vi "rsscope_core_global.vi"() -> ()   [LabVIEW 2018] (continued)
 Models"="", "Instrument Options"="K3", "Flags"=0, "Help"="Sets the LIN standard to search for CRC errors.\n\nAvailable Repeated Capabilities:\nNone\n\nRemote-control command(s):\nSEARch:TRIGger:LIN:STANdard"}, {"Level"=5, "Class Only"=FALSE, "Identifier"="RSSCOPE_ATTR_SEARCH_LIN_IDENTIFIER_PARITY_ERROR", "Descriptive Name"="Search LIN Identifier Parity Error", "Data Type"=3, "Command"="SEAR:TRIG:LIN:IPER", "Access"=2, "Range Table"="", "Read Callback"="rsscope_FormatSearchNameBoolean_ReadCallback.vi", "Write Callback"="rsscope_FormatSearchNameBoolean_WriteCallback.vi", "Supported Models"="", "Instrument Options"="K3", "Flags"=0, "Help"="Searches for errors in the identifier parity bits. These are the bits 6 and 7 of the identifier.\n\nAvailable Repeated Capabilities:\nNone\n\nRemote-control command(s):\nSEARch:TRIGger:LIN:IPERror"}, {"Level"=5, "Class Only"=FALSE, "Identifier"="RSSCOPE_ATTR_SEARCH_LIN_SYNC_ERROR", "Descriptive Name"="Search LIN Sync Error", "Data Type"=3, "Command"="SEAR:TRIG:LIN:SYER", "Access"=2, "Range Table"="", "Read Callback"="rsscope_FormatSearchNameBoolean_ReadCallback.vi", "Write Callback"="rsscope_FormatSearchNameBoolean_WriteCallback.vi", "Supported Models"="", "Instrument Options"="K3", "Flags"=0, "Help"="Searches for synchronization errors.\n\nAvailable Repeated Capabilities:\nNone\n\nRemote-control command(s):\nSEARch:TRIGger:LIN:SYERror"}, {"Level"=4, "Class Only"=TRUE, "Identifier"="", "Descriptive Name"="Results", "Data Type"=0, "Command"="", "Access"=0, "Range Table"="", "Read Callback"="", "Write Callback"="", "Supported Models"="", "Instrument Options"="", "Flags"=0, "Help"="Returns the search result of the specified frame."}, {"Level"=5, "Class Only"=FALSE, "Identifier"="RSSCOPE_ATTR_SEARCH_LIN_SELECTED_FRAME", "Descriptive Name"="Search LIN Selected Frame", "Data Type"=0, "Command"="", "Access"=2, "Range Table"="", "Read Callback"="", "Write Callback"="", "Supported Models"="", "Instrument Options"="", "Flags"=0, "Help"="Sets the selector for the Frame repeated capability.\n\nAvailable Repeated Capabilities:\nNone\n\nRemote-control command(s):\n"}, {"Level"=5, "Class Only"=FALSE, "Identifier"="RSSCOPE_ATTR_SEARCH_LIN_FRAME_COUNT", "Descriptive Name"="Search LIN Frame Count", "Data Type"=0, "Command"="SEAR:RES:LIN:FCO?", "Access"=0, "Range Table"="", "Read Callback"="rsscope_FormatSearchNameInt32_ReadCallback.vi", "Write Callback"="", "Supported Models"="", "Instrument Options"="K3", "Flags"=0, "Help"="Returns the frame count for the selected serial bus.\n\nAvailable Repeated Capabilities:\nNone\n\nRemote-control command(s):\nSEARch:RESult:LIN:FCOunt?"}, {"Level"=5, "Class Only"=FALSE, "Identifier"="RSSCOPE_ATTR_SEARCH_LIN_FRAME_SYMBOLIC_DATA", "Descriptive Name"="Search LIN Frame Symbolic Data", "Data Type"=2, "Command"="SEAR:RES:LIN:FRAM<Frame>:SDAT?", "Access"=0, "Range Table"="", "Read Callback"="rsscope_FormatLINSearchNameFrameRepCapString_ReadCallback.vi", "Write Callback"="rsscope_FormatLINSearchNameFrameRepCapString_WriteCallback.vi", "Supported Models"="", "Instrument Options"="", "Flags"=0, "Help"="Returns the symbolic data of the frame.\n\nAvailable Repeated Capabilities:\nNone\n\nRemote-control command(s):\nSEARch:RESult:LIN:FRAMe<m>:SDATa?"}, {"Level"=5, "Class Only"=FALSE, "Identifier"="RSSCOPE_ATTR_SEARCH_LIN_FRAME_SYMBOLIC_DATA_EXPORT", "Descriptive Name"="Search LIN Frame Symbolic Data Export", "Data Type"=2, "Command"="SEAR:RES:LIN:FRAM<Frame>:SDEX?", "Access"=0, "Range Table"="", "Read Callback"="rsscope_FormatLINSearchNameFrameRepCapString_ReadCallback.vi", "Write Callback"="rsscope_FormatLINSearchNameFrameRepCapString_WriteCallback.vi", "Supported Models"="", "Instrument Options"="", "Flags"=0, "Help"="Returns the symbolic data of the frame for the export format.\n\nAvailable Repeated Capabilities:\nNone\n\nRemote-control command(s):\nSEARch:RESult:LIN:FRAMe<m>:SDEXport?"}, {"Level"=3, "Class Only"=TRUE, "Identifier"="", "Descriptive Name"="CAN", "Data Type"=0, "Command"="", "Access"=0, "Range Table"="", "Read Callback"="", "Write Callback"="", "Supported Models"="", "Instrument Options"="", "Flags"=0, "Help"="Search decoded data in CAN protocol."}, {"Level"=4, "Class Only"=FALSE, "Identifier"="RSSCOPE_ATTR_SEARCH_CAN_ENABLED", "Descriptive Name"="Search CAN Enabled", "Data Type"=3, "Command"="SEAR:TRIG:CAN", "Access"=2, "Range Table"="", "Read Callback"="rsscope_FormatSearchNameBoolean_ReadCallback.vi", "Write Callback"="rsscope_FormatSearchNameBoolean_WriteCallback.vi", "Supported Models"="", "Instrument Options"="", "Flags"=0, "Help"="Includes the search conditions for the CAN trigger event type in the next search.\n\nAvailable Repeated Capabilities:\nNone\n\nRemote-control command(s):\nSEARch:TRIGger:CAN[:STATe]"}, {"Level"=4, "Class Only"=FALSE, "Identifier"="RSSCOPE_ATTR_SEARCH_CAN_COPY_FROM_A", "Descriptive Name"="Search CAN Copy From A", "Data Type"=2, "Command"="SEAR:TRIG:CAN:ACOP", "Access"=1, "Range Table"="", "Read Callback"="", "Write Callback"="", "Supported Models"="", "Instrument Options"="", "Flags"=0, "Help"="Copies the trigger event configuration from Trigger A for the selcted CAN bus to the search condition settings.\n\nAvailable Repeated Capabilities:\nNone\n\nRemote-control command(s):\nSEARch:TRIGger:CAN:ACOPy"}, {"Level"=4, "Class Only"=FALSE, "Identifier"="RSSCOPE_ATTR_SEARCH_CAN_START_OF_FRAME_ENABLED", "Descriptive Name"="Search CAN Start Of Frame Enabled", "Data Type"=3, "Command"="SEAR:TRIG:CAN:SSOF", "Access"=2, "Range Table"="", "Read Callback"="rsscope_FormatSearchNameBoolean_ReadCallback.vi", "Write Callback"="rsscope_FormatSearchNameBoolean_WriteCallback.vi", "Supported Models"="", "Instrument Options"="", "Flags"=0, "Help"="Enables the search for a start of frame.\n\nAvailable Repeated Capabilities:\nNone\n\nRemote-control command(s):\nSEARch:TRIGger:CAN[:SSOFrame]"}, {"Level"=4, "Class Only"=FALSE, "Identifier"="RSSCOPE_ATTR_SEARCH_CAN_FRAME_TYPE_ENABLED", "Descriptive Name"="Search CAN Frame Type Enabled", "Data Type"=3, "Command"="SEAR:TRIG:CAN:SFTY", "Access"=2, "Range Table"="", "Read Callback"="rsscope_FormatSearchNameBoolean_ReadCallback.vi", "Write Callback"="rsscope_FormatSearchNameBoolean_WriteCallback.vi", "Supported Models"="", "Instrument Options"="", "Flags"=0, "Help"="Enables the search for a specified frame type.\n\nAvailable Repeated Capabilities:\nNone\n\nRemote-control command(s):\nSEARch:TRIGger:CAN:SFTYpe"}, {"Level"=4, "Class Only"=FALSE, "Identifier"="RSSCOPE_ATTR_SEARCH_CAN_FRAME_IDENTIFIER_ENABLED", "Descriptive Name"="Search CAN Frame Identifier Enabled", "Data Type"=3, "Command"="SEAR:TRIG:CAN:SFID", "Access"=2, "Range Table"="", "Read Callback"="rsscope_FormatSearchNameBoolean_ReadCallback.vi", "Write Callback"="rsscope_FormatSearchNameBoolean_WriteCallback.vi", "Supported Models"="", "Instrument Options"="", "Flags"=0, "Help"="Enables the search for frame indentifier.\n\nAvailable Repeated Capabilities:\nNone\n\nRemote-control command(s):\nSEARch:TRIGger:CAN:SFIDentifier"}, {"Level"=4, "Class Only"=FALSE, "Identifier"="RSSCOPE_ATTR_SEARCH_CAN_IDENTIFIER_DATA_ENABLED", "Descriptive Name"="Search CAN Identifier Data Enabled", "Data Type"=3, "Command"="SEAR:TRIG:CAN:SIDD", "Access"=2, "Range Table"="", "Read Callback"="rsscope_FormatSearchNameBoolean_ReadCallback.vi", "Write Callback"="rsscope_FormatSearchNameBoolean_WriteCallback.vi", "Supported Models"="", "Instrument Options"="", "Flags"=0, "Help"="Enables the search for identifier and data.\n\nAvailable Repeated Capabilities:\nNone\n\nRemote-control command(s):\nSEARch:TRIGger:CAN:SIDData"}, {"Level"=4, "Class Only"=FALSE, "Identifier"="RSSCOPE_ATTR_SEARCH_CAN_SYMBOLIC_ENABLED", "Descriptive Name"="Search CAN Symbolic Enabled", "Data Type"=3, "Command"="SEAR:TRIG:CAN:SSYM", "Access"=2, "Range Table"="", "Read Callback"="rsscope_FormatSearchNameBoolean_ReadCallback.vi", "Write Callback"="rsscope_FormatSearchNameBoolean_WriteCallback.vi", "Supported Models"="", "Instrument Options"="", "Flags"=0, "Help"="Enables the symbolic search and disables all other search criteria.\n\nAvailable Repeated Capabilities:\nNone\n\nRemote-control command(s):\nSEARch:TRIGger:CAN:SSYMbolic"}, {"Level"=4, "Class Only"=FALSE, "Identifier"="RSSCOPE_ATTR_SEARCH_CAN_FRAME_TYPE", "Descriptive Name"="Search CAN Frame Type", "Data Type"=0, "Command"="SEAR:TRIG:CAN:FTYP", "Access"=2, "Range Table"="rsscope_rngProtocolCANTriggFrameType", "Read Callback"="rsscope_FormatSearchNameInt32_ReadCallback.vi", "Write Callback"="rsscope_FormatSearchNameInt32_WriteCallback.vi", "Supported Models"="", "Instrument Options"="", "Flags"=0, "Help"="Selects the CAN frame type to be searched for.\n\nAvailable Repeated Capabilities:\nNone\n\nRemote-control command(s):\nSEARch:TRIGger:CAN:FTYPe"}, {"Level"=4, "Class Only"=FALSE, "Identifier"="RSSCOPE_ATTR_SEARCH_CAN_STANDARD", "Descriptive Name"="Search CAN Standard", "Data Type"=0, "Command"="SEAR:TRIG:CAN:FDAT:STAN", "Access"=2, "Range Table"="rsscope_rngCANStandard", "Read Callback"="rsscope_FormatSearchNameInt32_ReadCallback.vi", "Write Callback"="rsscope_FormatSearchNameInt32_WriteCallback.vi", "Supported Models"="", "Instrument Options"="K9", "Flags"=0, "Help"="Selects the CAN standard: CAN, CAN FD, or Any.\n\nAvailable Repeated Capabilities:\nNone\n\nRemote-control command(s):\nSEARch:TRIGger:CAN:FDATa:STANdard"}, {"Level"=4, "Class Only"=FALSE, "Identifier"="RSSCOPE_ATTR_SEARCH_CAN_ID_TYPE", "Descriptive Name"="Search CAN ID Type", "Data Type"=0, "Command"="SEAR:TRIG:CAN:ITYP", "Access"=2, "Range Table"="rsscope_rngProtocolCANIDType", "Read Callback"="rsscope_FormatSearchNameInt32_ReadCallback.vi", "Write Callback"="rsscope_FormatSearchNameInt32_WriteCallback.vi", "Supported Models"="", "Instrument Options"="", "Flags"=0, "Help"="Selects the format of data and remote frames: 11 bit for CAN base frames, or 29 bits for CAN extended frames.\n\nAvailable Repeated Capabilities:\nNone\n\nRemote-control command(s):\nSEARch:TRIGger:CAN:ITYPe"}, {"Level"=4, "Class Only"=FALSE, "Identifier"="RSSCOPE_ATTR_SEARCH_CAN_IDENTIFIER_CONDITION", "Descriptive Name"="Search CAN Identifier Condition", "Data Type"=0, "Command"="SEAR:TRIG:CAN:ICON", "Access"=2, "Range Table"="rsscope_rngProtocolTriggerCondition", "Read Callback"="rsscope_FormatSearchNameInt32_ReadCallback.vi", "Write Callback"="rsscope_FormatSearchNameInt32_WriteCallback.vi", "Supported Models"="", "Instrument Options"="", "Flags"=0, "Help"="Sets the operator to set a specific identifier or an identifier range.\n\nAvailable Repeated Capabilities:\nNone\n\nRemote-control command(s):\nSEARch:TRIGger:CAN:ICONdition"}, {"Level"=4, "Class Only"=FALSE, "Identifier"="RSSCOPE_ATTR_SEARCH_CAN_IDENTIFIER_MIN", "Descriptive Name"="Search CAN Identifier Min", "Data Type"=2, "Command"="SEAR:TRIG:CAN:IMIN", "Access"=1, "Range Table"="", "Read Callback"="", "Write Callback"="rsscope_FormatSearchNameString_WriteCallback.vi", "Supported Models"="", "Instrument Options"="", "Flags"=0, "Help"="Specifies a message identifier pattern, or sets the start value of an identifier range.\n\nAvailable Repeated Capabilities:\nNone\n\nRemote-control command(s):\nSEARch:TRIGger:CAN:IMIN"}, {"Level"=4, "Class Only"=FALSE, "Identifier"="RSSCOPE_ATTR_SEARCH_CAN_IDENTIFIER_MAX", "Descriptive Name"="Search CAN Identifier Max", "Data Type"=2, "Command"="SEAR:TRIG:CAN:IMAX", "Access"=1, "Range Table"="", "Read Callback"="", "Write Callback"="rsscope_FormatSearchNameString_WriteCallback.vi", "Supported Models"="", "Instrument Options"="", "Flags"=0, "Help"="Sets the end value of an identifier range if RSSCOPE_ATTR_SEARCH_CAN_IDENTIFIER_CONDITION is set to In range or Out of range.\n\nAvailable Repeated Capabilities:\nNone\n\nRemote-control command(s):\nSEARch:TRIGger:CAN:IMAX"}, {"Level"=4, "Class Only"=FALSE, "Identifier"="RSSCOPE_ATTR_SEARCH_CAN_FD_BITS_FDF", "Descriptive Name"="Search CAN FD Bits FDF", "Data Type"=0, "Command"="SEAR:TRIG:CAN:FDAT", "Access"=2, "Range Table"="rsscope_rngCANFDBits", "Read Callback"="rsscope_FormatSearchNameInt32_ReadCallback.vi", "Write Callback"="rsscope_FormatSearchNameInt32_WriteCallback.vi", "Supported Models"="", "Instrument Options"="K9", "Flags"=0, "Help"="Specifies the CAN FD frame format. It corresponds to the EDL bit (extended data length), which only exists in CAN FD format.\n\nAvailable Repeated Capabilities:\nNone\n\nRemote-control command(s):\nSEARch:TRIGger:CAN:FDATa[:FDF]"}, {"Level"=4, "Class Only"=FALSE, "Identifier"="RSSCOPE_ATTR_SEARCH_CAN_FD_BITS_BRS", "Descriptive Name"="Search CAN FD Bits BRS", "Data Type"=0, "Command"="SEAR:TRIG:CAN:FDAT:BRS", "Access"=2, "Range Table"="rsscope_rngCANFDBits", "Read Callback"="rsscope_FormatSearchNameInt32_ReadCallback.vi", "Write Callback"="rsscope_FormatSearchNameInt32_WriteCallback.vi", "Supported Models"="", "Instrument Options"="K9", "Flags"=0, "Help"="Sets the bit rate switch bit.\n\nAvailable Repeated Capabilities:\nNone\n\nRemote-control command(s):\nSEARch:TRIGger:CAN:FDATa:BRS"}, {"Level"=4, "Class Only"=FALSE, "Identifier"="RSSCOPE_ATTR_SEARCH_CAN_FD_BITS_ESI", "Descriptive Name"="Search CAN FD Bits ESI", "Data Type"=0, "Command"="SEAR:TRIG:CAN:FDAT:ESI", "Access"=2, "Range Table"="rsscope_rngCANFDBits", "Read Callback"="rsscope_FormatSearchNameInt32_ReadCallback.vi", "Write Callback"="rsscope_FormatSearchNameInt32_WriteCallback.vi", "Supported Models"="", "Instrument Options"="K9", "Flags"=0, "Help"="Sets the error state indicator bit.\n\nAvailable Repeated Capabilities:\nNone\n\nRemote-control command(s):\nSEARch:TRIGger:CAN:FDATa:ESI"}, {"Level"=4, "Class Only"=FALSE, "Identifier"="RSSCOPE_ATTR_SEARCH_CAN_DLC_CONDITION", "Descriptive Name"="Search CAN DLC Condition", "Data Type"=0, "Command"="SEAR:TRIG:CAN:DLCC", "Access"=2, "Range Table"="rsscope_rngProtocolTriggerCondition", "Read Callback"="rsscope_FormatSearchNameInt32_ReadCallback.vi", "Write Callback"="rsscope_FormatSearchNameInt32_WriteCallback.vi", "Supported Models"="", "Instrument Options"="", "Flags"=0, "Help"="Operator to set the data length code for searching on CAN data. For big endian transfer direction, you can search for a number of bytes less than the DLC of the frame, that means, on the beginning of the data pattern. For little endian transfer direction, the exact number of data bytes in the frame must be set. The number of data bytes to be found is set with RSSCOPE_ATTR_SEARCH_CAN_DLC\n\nAvailable Repeated Capabilities:\nNone\n\nRemote-control command(s):\nSEARch:TRIGger:CAN:DLCCondition"}, {"Level"=4, "Class Only"=FALSE, "Identifier"="RSSCOPE_ATTR_SEARCH_CAN_DLC", "Descriptive Name"="Search CAN DLC", "Data Type"=0, "Command"="SEAR:TRIG:CAN:DLC", "Access"=2, "Range Table"="RsScope_rngSearchCANDLC", "Read Callback"="rsscope_FormatSearchNameInt32_ReadCallback.vi", "Write Callback"="rsscope_FormatSearchNameInt32_WriteCallback.vi", "Supported Models"="", "Instrument Options"="", "Flags"=0, "Help"="Sets the Data Length Code, the number of data bytes to be found. For complete definition, set also the operator with RSSCOPE_ATTR_SEARCH_CAN_DLC_CONDITION.\n\nAvailable Repeated Capabilities:\nNone\n\nRemote-control command(s):\nSEARch:TRIGger:CAN:DLC"}, {"Level"=4, "Class Only"=FALSE, "Identifier"="RSSCOPE_ATTR_SEARCH_CAN_POSITION_CONDITION", "Descriptive Name"="Search CAN Position Condition", "Data Type"=0, "Command"="SEAR:TRIG:CAN:FDAT:DPOP", "Access"=2, "Range Table"="rsscope_rngProtocolCANPositionCondition", "Read Callback"="rsscope_FormatSearchNameInt32_ReadCallback.vi", "Write Callback"="rsscope_FormatSearchNameInt32_WriteCallback.vi", "Supported Models"="", "Instrument Options"="K9", "Flags"=0, "Help"="Sets the operator to define an exact position or a data range where the instrument looks for the specified data pattern.\n\nAvailable Repeated Capabilities:\nNone\n\nRemote-control command(s):\nSEARch:TRIGger:CAN:FDATa:DPOPerator"}, {"Level"=4, "Class Only"=FALSE, "Identifier"="RSSCOPE_ATTR_SEARCH_CAN_POSITION_MIN", "Descriptive Name"="Search CAN Position Min", "Data Type"=0, "Command"="SEAR:TRIG:CAN:FDAT:DPOS", "Access"=2, "Range Table"="rsscope_rngCANPositionMin", "Read Callback"="rsscope_FormatSearchNameInt32_ReadCallback.vi", "Write Callback"="rsscope_FormatSearchNameInt32_WriteCallback.vi", "Supported Models"="", "Instrument Options"="K9", "Flags"=0, "Help"="Defines the first possible start position of the data pattern.\n\nAvailable Repeated Capabilities:\nNone\n\nRemote-control command(s):\nSEARch:TRIGger:CAN:FDATa:DPOSition"}, {"Level"=4, "Class Only"=FALSE, "Identifier"="RSSCOPE_ATTR_SEARCH_CAN_POSITION_MAX", "Descriptive Name"="Search CAN Position Max", "Data Type"=0, "Command"="SEAR:TRIG:CAN:FDAT:DPTO", "Access"=2, "Range Table"="rsscope_rngCANPositionMax", "Read Callback"="rsscope_FormatSearchNameInt32_ReadCallback.vi", "Write Callback"="rsscope_FormatSearchNameInt32_WriteCallback.vi", "Supported Models"="", "Instrument Options"="K9", "Flags"=0, "Help"="Defines the last possible start position of the data pattern if &apos;Condition&apos; is &apos;In range&apos; and &apos;Out of range&apos;.\n\nAvailable Repeated Capabilities:\nNone\n\nRemote-control command(s):\nSEARch:TRIGger:CAN:FDATa:DPTO"}, {"Level"=4, "Class Only"=FALSE, "Identifier"="RSSCOPE_ATTR_SEARCH_CAN_DATA_CONDITION", "Descriptive Name"="Search CAN Data Condition", "Data Type"=0, "Command"="SEAR:TRIG:CAN:DCON", "Access"=2, "Range Table"="rsscope_rngProtocolTriggerCondition", "Read Callback"="rsscope_FormatSearchNameInt32_ReadCallback.vi", "Write Callback"="rsscope_FormatSearchNameInt32_WriteCallback.vi", "Supported Models"="", "Instrument Options"="", "Flags"=0, "Help"="Sets the operator to set a specific data pattern or a data pattern range.\n\nAvailable Repeated Capabilities:\nNone\n\nRemote-control command(s):\nSEARch:TRIGger:CAN:DCONdition"}, {"Level"=4, "Class Only"=FALSE, "Identifier"="RSSCOPE_ATTR_SEARCH_CAN_DATA_MIN", "Descriptive Name"="Search CAN Data Min", "Data Type"=2, "Command"="SEAR:TRIG:CAN:DMIN", "Access"=1, "Range Table"="", "Read Callback"="", "Write Callback"="rsscope_FormatSearchNameString_WriteCallback.vi", "Supported Models"="", "Instrument Options"="", "Flags"=0, "Help"="Specifies a data pattern, or sets the start value of a data pattern range.\n\nAvailable Repeated Capabilities:\nNone\n\nRemote-control command(s):\nSEARch:TRIGger:CAN:DMIN"}, {"Level"=4, "Class Only"=FALSE, "Identifier"="RSSCOPE_ATTR_SEARCH_CAN_DATA_MAX", "Descriptive Name"="Search CAN Data Max", "Data Type"=2, "Command"="SEAR:TRIG:CAN:DMAX", "Access"=1, "Range Table"="", "Read Callback"="", "Write Callback"="rsscope_FormatSearchNameString_WriteCallback.vi", "Supported Models"="", "Instrument Options"="", "Flags"=0, "Help"="Sets the end value of an data range if RSSCOPE_ATTR_SEARCH_CAN_DATA_CONDITION is set to In range or Out of range.\n\nAvailable Repeated Capabilities:\nNone\n\nRemote-control command(s):\nSEARch:TRIGger:CAN:DMAX"}, {"Level"=4, "Class Only"=FALSE, "Identifier"="RSSCOPE_ATTR_SEARCH_CAN_CRC_ERROR", "Descriptive Name"="Search CAN CRC Error", "Data Type"=3, "Command"="SEAR:TRIG:CAN:CRC", "Access"=2, "Range Table"="", "Read Callback"="rsscope_FormatSearchNameBoolean_ReadCallback.vi", "Write Callback"="rsscope_FormatSearchNameBoolean_WriteCallback.vi", "Supported Models"="", "Instrument Options"="", "Flags"=0, "Help"="Searches for errors in the Cyclic Redundancy Check.\n\nAvailable Repeated Capabilities:\nNone\n\nRemote-control command(s):\nSEARch:TRIGger:CAN:CRCerror"}, {"Level"=4, "Class Only"=FALSE, "Identifier"="RSSCOPE_ATTR_SEARCH_CAN_BIT_STUFFING_ERROR", "Descriptive Name"="Search CAN Bit Stuffing Error", "Data Type"=3, "Command"="SEAR:TRIG:CAN:BITS", "Access"=2, "Range Table"="", "Read Callback"="rsscope_FormatSearchNameBoolean_ReadCallback.vi", "Write Callback"="rsscope_FormatSearchNameBoolean_WriteCallback.vi", "Supported Models"="", "Instrument Options"="", "Flags"=0, "Help"="Searches for bit stuffing errors.\n\nAvailable Repeated Capabilities:\nNone\n\nRemote-control command(s):\nSEARch:TRIGger:CAN:BITSterror"}, {"Level"=4, "Class Only"=FALSE, "Identifier"="RSSCOPE_ATTR_SEARCH_CAN_ACK_ERROR", "Descriptive Name"="Search CAN Ack Error", "Data Type"=3, "Command"="SEAR:TRIG:CAN:ACK", "Access"=2, "Range Table"="", "Read Callback"="rsscope_FormatSearchNameBoolean_ReadCallback.vi", "Write Callback"="rsscope_FormatSearchNameBoolean_WriteCallback.vi", "Supported Models"="", "Instrument Options"="", "Flags"=0, "Help"="Searches for acknowledgement errors. An acknowledgement error occurs when the transmitter does not receive an acknowledgment - a dominant bit during the Ack Slot.\n\nAvailable Repeated Capabilities:\nNone\n\nRemote-control command(s):\nSEARch:TRIGger:CAN:ACKerror"}, {"Level"=4, "Class Only"=FALSE, "Identifier"="RSSCOPE_ATTR_SEARCH_CAN_STUFF_COUNT_ERROR", "Descriptive Name"="Search CAN Stuff Count Error", "Data Type"=3, "Command"="SEAR:TRIG:CAN:FDAT:SCER", "Access"=2, "Range Table"="", "Read Callback"="rsscope_FormatSearchNameBoolean_ReadCallback.vi", "Write Callback"="rsscope_FormatSearchNameBoolean_WriteCallback.vi", "Supported Models"="", "Instrument Options"="K3", "Flags"=0, "Help"="Triggers on stuff count errors. A stuff count error occurs if th received stuff count value does not match the value calculated from the own stuff bit count.\n\nAvailable Repeated Capabilities:\nNone\n\nRemote-control command(s):\nSEARch:TRIGger:CAN:FDATa:SCERror"}, {"Level"=4, "Class Only"=TRUE, "Identifier"="", "Descriptive Name"="Symbolic", "Data Type"=0, "Command"="", "Access"=0, "Range Table"="", "Read Callback"="", "Write Callback"="", "Supported Models"="", "Instrument Options"="", "Flags"=0, "Help"="This class configures symbolic trigger."}, {"Level"=5, "Class Only"=FALSE, "Identifier"="RSSCOPE_ATTR_SEARCH_CAN_SYMBOLIC_MESSAGE", "Descriptive Name"="Search CAN Symbolic Message", "Data Type"=2, "Command"="SEAR:TRIG:CAN:SYMB:MSGV", "Access"=2, "Range Table"="", "Read Callback"="rsscope_FormatSearchNameString_ReadCallback.vi", "Write Callback"="rsscope_FormatSearchNameString_WriteCallback.vi", "Supported Models"="", "Instrument Options"="", "Flags"=0, "Help"="Sets the message to be triggered or searched for.\n\nAvailable Repeated Capabilities:\nNone\n\nRemote-control command(s):\nSEARch:TRIGger:CAN:SYMBolic:MSGValue"}, {"Level"=5, "Class Only"=FALSE, "Identifier"="RSSCOPE_ATTR_SEARCH_CAN_SYMBOLIC_SEARCH_FOR_SIGNAL", "Descriptive Name"="Search CAN Symbolic Search For Signal", "Data Type"=3, "Command"="SEAR:TRIG:CAN:SYMB:SSIG", "Access"=2, "Range Table"="", "Read Callback"="rsscope_FormatSearchNameBoolean_ReadCallback.vi", "Write Callback"="rsscope_FormatSearchNameBoolean_WriteCallback.vi", "Supported Models"="", "Instrument Options"="", "Flags"=0, "Help"="Enables the search for a specific signal value that is part of the selected message.\n\nAvailable Repeated Capabilities:\nNone\n\nRemote-control command(s):\nSEARch:TRIGger:CAN:SYMBolic:SSIGnals"}, {"Level"=5, "Class Only"=FALSE, "Identifier"="RSSCOPE_ATTR_SEARCH_CAN_SYMBOLIC_SIGNAL_VALUE", "Descriptive Name"="Search CAN Symbolic Signal Value", "Data Type"=2, "Command"="SEAR:TRIG:CAN:SYMB:SIGV", "Access"=2, "Range Table"="", "Read Callback"="rsscope_FormatSearchNameString_ReadCallback.vi", "Write Callback"="rsscope_FormatSearchNameString_WriteCallback.vi", "Supported Models"="", "Instrument Options"="", "Flags"=0, "Help"="Sets the signal name to be triggered or searched for.\n\nAvailable Repeated Capabilities:\nNone\n\nRemote-control command(s):\nSEARch:TRIGger:CAN:SYMBolic:SIGValue"}, {"Level"=5, "Class Only"=FALSE, "Identifier"="RSSCOPE_ATTR_SEARCH_CAN_SYMBOLIC_SIGNAL_MIN", "Descriptive Name"="Search CAN Symbolic Signal Min", "Data Type"=1, "Command"="SEAR:TRIG:CAN:SYMB:DMIN", "Access"=2, "Range Table"="", "Read Callback"="rsscope_FormatSearchNameReal64_ReadCallback.vi", "Write Callback"="rsscope_FormatSearchNameReal64_WriteCallback.vi", "Supported Models"="", "Instrument Options"="", "Flags"=0, "Help"="Defines the minimum data value of the signal.\n\nAvailable Repeated Capabilities:\nNone\n\nRemote-control command(s):\nSEARch:TRIGger:CAN:SYMBolic:DMIN"}, {"Level"=5, "Class Only"=FALSE, "Identifier"="RSSCOPE_ATTR_SEARCH_CAN_SYMBOLIC_SIGNAL_MAX", "Descriptive Name"="Search CAN Symbolic Signal Max", "Data Type"=1, "Command"="SEAR:TRIG:CAN:SYMB:DMAX", "Access"=2, "Range Table"="", "Read Callback"="rsscope_FormatSearchNameReal64_ReadCallback.vi", "Write Callback"="rsscope_FormatSearchNameReal64_WriteCallback.vi", "Supported Models"="", "Instrument Options"="", "Flags"=0, "Help"="Defines the maximum data value of the signal. This value is required to specify a range if condition is &apos;In range&apos; or &apos;Out of range&apos;.\n\nAvailable Repeated Capabilities:\nNone\n\nRemote-control command(s):\nSEARch:TRIGger:CAN:SYMBolic:DMAX"}, {"Level"=5, "Class Only"=FALSE, "Identifier"="RSSCOPE_ATTR_SEARCH_CAN_SYMBOLIC_SIGNAL_ENUM_VALUE", "Descriptive Name"="Search CAN Symbolic Signal Enum Value", "Data Type"=0, "Command"="SEAR:TRIG:CAN:SYMB:SGEV", "Access"=2, "Range Table"="", "Read Callback"="rsscope_FormatSearchNameInt32_ReadCallback.vi", "Write Callback"="rsscope_FormatSearchNameInt32_WriteCallback.vi", "Supported Models"="", "Instrument Options"="", "Flags"=0, "Help"="Sets a symbolic data value for signals with enumerated values.\n\nAvailable Repeated Capabilities:\nNone\n\nRemote-control command(s):\nSEARch:TRIGger:CAN:SYMBolic:SGEValue"}, {"Level"=3, "Class Only"=TRUE, "Identifier"="", "Descriptive Name"="FlexRay", "Data Type"=0, "Command"="", "Access"=0, "Range Table"="", "Read Callback"="", "Write Callback"="", "Supported Models"="", "Instrument Options"="", "Flags"=0, "Help"="Search decoded data in FlexRay protocol."}, {"Level"=4, "Class Only"=FALSE, "Identifier"="RSSCOPE_ATTR_SEARCH_FLEXRAY_ENABLED", "Descriptive Name"="Search FlexRay Enabled", "Data Type"=3, "Command"="SEAR:TRIG:FLXR", "Access"=2, "Range Table"="", "Read Callback"="rsscope_FormatSearchNameBoolean_ReadCallback.vi", "Write Callback"="rsscope_FormatSearchNameBoolean_WriteCallback.vi", "Supported Models"="", "Instrument Options"="", "Flags"=0, "Help"="Includes the search conditions for the FlexRay trigger event type in the next search.\n\nAvailable Repeated Capabilities:\nNone\n\nRemote-control command(s):\nSEARch:TRIGger:FLXRay[:STATe]"}, {"Level"=4, "Class Only"=FALSE, "Identifier"="RSSCOPE_ATTR_SEARCH_FLEXRAY_COPY_FROM_A", "Descriptive Name"="Search FlexRay Copy From A", "Data Type"=2, "Command"="SEAR:TRIG:FLXR:ACOP", "Access"=2, "Range Table"="", "Read Callback"="", "Write Callback"="", "Supported Models"="", "Instrument Options"="", "Flags"=0, "Help"="Copies the trigger event configuration from Trigger A for the selected FlexRay bus to the search condition settings.\n\nAvailable Repeated Capabilities:\nNone\n\nRemote-control command(s):\nSEARch:TRIGger:FLXRay:ACOPy"}, {"Level"=4, "Class Only"=FALSE, "Identifier"="RSSCOPE_ATTR_SEARCH_FLEXRAY_START_OF_FRAME_ENABLED", "Descriptive Name"="Search FlexRay Start Of Frame Enabled", "Data Type"=3, "Command"="SEAR:TRIG:FLXR:SSOF", "Access"=2, "Range Table"="", "Read Callback"="rsscope_FormatSearchNameBoolean_ReadCallback.vi", "Write Callback"="rsscope_FormatSearchNameBoolean_WriteCallback.vi", "Supported Models"="", "Instrument Options"="", "Flags"=0, "Help"="Enables the search for a start of frame.\n\nAvailable Repeated Capabilities:\nNone\n\nRemote-control command(s):\nSEARch:TRIGger:FLXRay[:SSOFrame]"}, {"Level"=4, "Class Only"=FALSE, "Identifier"="RSSCOPE_ATTR_SEARCH_FLEXRAY_SYMBOL_ENABLED", "Descriptive Name"="Search FlexRay Symbol Enabled", "Data Type"=3, "Command"="SEAR:TRIG:FLXR:SSYM", "Access"=2, "Range Table"="", "Read Callback"="rsscope_FormatSearchNameBoolean_ReadCallback.vi", "Write Callback"="rsscope_FormatSearchNameBoolean_WriteCallback.vi", "Supported Models"="", "Instrument Options"="", "Flags"=0, "Help"="Enables the search for specified symbol.\n\nAvailable Repeated Capabilities:\nNone\n\nRemote-control command(s):\nSEARch:TRIGger:FLXRay:SSYMbol"}, {"Level"=4, "Class Only"=FALSE, "Identifier"="RSSCOPE_ATTR_SEARCH_FLEXRAY_IDENTIFIER_DATA_ENABLED", "Descriptive Name"="Search FlexRay Identifier Data Enabled", "Data Type"=3, "Command"="SEAR:TRIG:FLXR:SIDD", "Access"=2, "Range Table"="", "Read Callback"="rsscope_FormatSearchNameBoolean_ReadCallback.vi", "Write Callback"="rsscope_FormatSearchNameBoolean_WriteCallback.vi", "Supported Models"="", "Instrument Options"="", "Flags"=0, "Help"="Enables the search for indentifier and data.\n\nAvailable Repeated Capabilities:\nNone\n\nRemote-control command(s):\nSEARch:TRIGger:FLXRay:SIDData"}, {"Level"=4, "Class Only"=FALSE, "Identifier"="RSSCOPE_ATTR_SEARCH_FLEXRAY_ERROR_CONDITION_ENABLED", "Descriptive Name"="Search FlexRay Error Condition Enabled", "Data Type"=3, "Command"="SEAR:TRIG:FLXR:SERR", "Access"=2, "Range Table"="", "Read Callback"="rsscope_FormatSearchNameBoolean_ReadCallback.vi", "Write Callback"="rsscope_FormatSearchNameBoolean_WriteCallback.vi", "Supported Models"="", "Instrument Options"="", "Flags"=0, "Help"="Enables the search for specified error or error combination.\n\nAvailable Repeated Capabilities:\nNone\n\nRemote-control command(s):\nSEARch:TRIGger:FLXRay:SERRor"}, {"Level"=4, "Class Only"=FALSE, "Identifier"="RSSCOPE_ATTR_SEARCH_FLEXRAY_PAYLOAD_PREAMBLE", "Descriptive Name"="Search FlexRay Payload Preamble", "Data Type"=0, "Command"="SEAR:TRIG:FLXR:PLPR", "Access"=2, "Range Table"="rsscope_rngFlexRayIndicatorBits", "Read Callback"="rsscope_FormatSearchNameInt32_ReadCallback.vi", "Write Callback"="rsscope_FormatSearchNameInt32_WriteCallback.vi", "Supported Models"="", "Instrument Options"="", "Flags"=0, "Help"="Searches for the payload preamble indicator bit that indicates a Network Management Vector in the payload segment.\n\nAvailable Repeated Capabilities:\nNone\n\nRemote-control command(s):\nSEARch:TRIGger:FLXRay:PLPReamble"}, {"Level"=4, "Class Only"=FALSE, "Identifier"="RSSCOPE_ATTR_SEARCH_FLEXRAY_NULL_FRAME", "Descriptive Name"="Search FlexRay Null Frame", "Data Type"=0, "Command"="SEAR:TRIG:FLXR:NUFR", "Access"=2, "Range Table"="rsscope_rngFlexRayIndicatorBits", "Read Callback"="rsscope_FormatSearchNameInt32_ReadCallback.vi", "Write Callback"="rsscope_FormatSearchNameInt32_WriteCallback.vi", "Supported Models"="", "Instrument Options"="", "Flags"=0, "Help"="Searches for the null frame indicator bit, a frame without usable data.\n\nAvailable Repeated Capabilities:\nNone\n\nRemote-control command(s):\nSEARch:TRIGger:FLXRay:NUFRame"}, {"Level"=4, "Class Only"=FALSE, "Identifier"="RSSCOPE_ATTR_SEARCH_FLEXRAY_SYNC_FRAME", "Descriptive Name"="Search FlexRay Sync Frame", "Data Type"=0, "Command"="SEAR:TRIG:FLXR:SYFR", "Access"=2, "Range Table"="rsscope_rngFlexRayIndicatorBits", "Read Callback"="rsscope_FormatSearchNameInt32_ReadCallback.vi", "Write Callback"="rsscope_FormatSearchNameInt32_WriteCallback.vi", "Supported Models"="", "Instrument Options"="", "Flags"=0, "Help"="Searches for the sync frame used for synchronization of the FlexRay system. Only sync nodes can send this frame type.\n\nAvailable Repeated Capabilities:\nNone\n\nRemote-control command(s):\nSEARch:TRIGger:FLXRay:SYFRame"}, {"Level"=4, "Class Only"=FALSE, "Identifier"="RSSCOPE_ATTR_SEARCH_FLEXRAY_STARTUP_FRAME", "Descriptive Name"="Search FlexRay Startup Frame", "Data Type"=0, "Command"="SEAR:TRIG:FLXR:STFR", "Access"=2, "Range Table"="rsscope_rngFlexRayIndicatorBits", "Read Callback"="rsscope_FormatSearchNameInt32_ReadCallback.vi", "Write Callback"="rsscope_FormatSearchNameInt32_WriteCallback.vi", "Supported Models"="", "Instrument Options"="", "Flags"=0, "Help"="Searches for startup frames used for startup of the network. Only specific start nodes can send this frame type.\n\nAvailable Repeated Capabilities:\nNone\n\nRemote-control command(s):\nSEARch:TRIGger:FLXRay:STFRame"}, {"Level"=4, "Class Only"=FALSE, "Identifier"="RSSCOPE_ATTR_SEARCH_FLEXRAY_FRAME_ID_CONDITION", "Descriptive Name"="Search FlexRay Frame ID Condition", "Data Type"=0, "Command"="SEAR:TRIG:FLXR:FCON", "Access"=2, "Range Table"="rsscope_rngFlexRayCondition", "Read Callback"="rsscope_FormatSearchNameInt32_ReadCallback.vi", "Write Callback"="rsscope_FormatSearchNameInt32_WriteCallback.vi", "Supported Models"="", "Instrument Options"="", "Flags"=0, "Help"="Sets the operator to set a frame ID or a frame ID range.\n\nAvailable Repeated Capabilities:\nNone\n\nRemote-control command(s):\nSEARch:TRIGger:FLXRay:FCONdition"}, {"Level"=4, "Class Only"=FALSE, "Identifier"="RSSCOPE_ATTR_SEARCH_FLEXRAY_FRAME_ID_MIN", "Descriptive Name"="Search FlexRay Frame ID Min", "Data Type"=2, "Command"="SEAR:TRIG:FLXR:FMIN", "Access"=2, "Range Table"="", "Read Callback"="rsscope_FormatSearchNameString_ReadCallback.vi", "Write Callback"="rsscope_FormatSearchNameString_WriteCallback.vi", "Supported Models"="", "Instrument Options"="", "Flags"=0, "Help"="Specifies a frame identifier pattern - the number of the slot - or sets the start value of an identifier range.\n\nAvailable Repeated Capabilities:\nNone\n\nRemote-control command(s):\nSEARch:TRIGger:FLXRay:FMIN"}, {"Level"=4, "Class Only"=FALSE, "Identifier"="RSSCOPE_ATTR_SEARCH_FLEXRAY_FRAME_ID_MAX", "Descriptive Name"="Search FlexRay Frame ID Max", "Data Type"=2, "Command"="SEAR:TRIG:FLXR:FMAX", "Access"=2, "Range Table"="", "Read Callback"="rsscope_FormatSearchNameString_ReadCallback.vi", "Write Callback"="rsscope_FormatSearchNameString_WriteCallback.vi", "Supported Models"="", "Instrument Options"="", "Flags"=0, "Help"="Sets the end value of an identifier range if the condition RSSCOPE_ATTR_SEARCH_FLEXRAY_FRAME_ID_CONDITION is set to In range or Out of range.\n\nAvailable Repeated Capabilities:\nNone\n\nRemote-control command(s):\nSEARch:TRIGger:FLXRay:FMAX"}, {"Level"=4, "Class Only"=FALSE, "Identifier"="RSSCOPE_ATTR_SEARCH_FLEXRAY_PAYLOAD_LENGTH_CONDITION", "Descriptive Name"="Search FlexRay Payload Length Condition", "Data Type"=0, "Command"="SEAR:TRIG:FLXR:PCON", "Access"=2, "Range Table"="rsscope_rngFlexRayCondition", "Read Callback"="rsscope_FormatSearchNameInt32_ReadCallback.vi", "Write Callback"="rsscope_FormatSearchNameInt32_WriteCallback.vi", "Supported Models"="", "Instrument Options"="", "Flags"=0, "Help"="Sets the operator for the payload length search setting. You can defined an exact value, or a range.\n\nAvailable Repeated Capabilities:\nNone\n\nRemote-control command(s):\nSEARch:TRIGger:FLXRay:PCONdition"}, {"Level"=4, "Class Only"=FALSE, "Identifier"="RSSCOPE_ATTR_SEARCH_FLEXRAY_PAYLOAD_LENGTH_MIN", "Descriptive Name"="Search FlexRay Payload Length Min", "Data Type"=0, "Command"="SEAR:TRIG:FLXR:PMIN", "Access"=2, "Range Table"="rsscope_rngFlexRayPayloadMinMax", "Read Callback"="rsscope_FormatSearchNameInt32_ReadCallback.vi", "Write Callback"="rsscope_FormatSearchNameInt32_WriteCallback.vi", "Supported Models"="", "Instrument Options"="", "Flags"=0, "Help"="Specifies a payload length - the number of words in the payload segment - or sets the start value of an payload length range. Information is transmitted in 2-byte words, so the number of data bytes in the payload segment is twice the payload length.\n\nAvailable Repeated Capabilities:\nNone\n\nRemote-control command(s):\nSEARch:TRIGger:FLXRay:PMIN"}, {"Level"=4, "Class Only"=FALSE, "Identifier"="RSSCOPE_ATTR_SEARCH_FLEXRAY_PAYLOAD_LENGTH_MAX", "Descriptive Name"="Search FlexRay Payload Length Max", "Data Type"=0, "Command"="SEAR:TRIG:FLXR:PMAX", "Access"=2, "Range Table"="rsscope_rngFlexRayPayloadMinMax", "Read Callback"="rsscope_FormatSearchNameInt32_ReadCallback.vi", "Write Callback"="rsscope_FormatSearchNameInt32_WriteCallback.vi", "Supported Models"="", "Instrument Options"="", "Flags"=0, "Help"="Sets the end value of a payload length range if the condition RSSCOPE_ATTR_SEARCH_FLEXRAY_PAYLOAD_LENGTH_CONDITION is set to In range or Out of range.\n\nAvailable Repeated Capabilities:\nNone\n\nRemote-control command(s):\nSEARch:TRIGger:FLXRay:PMAX"}, {"Level"=4, "Class Only"=FALSE, "Identifier"="RSSCOPE_ATTR_SEARCH_FLEXRAY_CYCLE_COUNT_CONDITION", "Descriptive Name"="Search FlexRay Cycle Count Condition", "Data Type"=0, "Command"="SEAR:TRIG:FLXR:CEN", "Access"=2, "Range Table"="rsscope_rngFlexRayCondition", "Read Callback"="rsscope_FormatSearchNameInt32_ReadCallback.vi", "Write Callback"="rsscope_FormatSearchNameInt32_WriteCallback.vi", "Supported Models"="", "Instrument Options"="", "Flags"=0, "Help"="Sets the operator to define a cycle count or a cycle count range.\n\nAvailable Repeated Capabilities:\nNone\n\nRemote-control command(s):\nSEARch:TRIGger:FLXRay:CENable"}, {"Level"=4, "Class Only"=FALSE, "Identifier"="RSSCOPE_ATTR_SEARCH_FLEXRAY_CYCLE_COUNT_MIN", "Descriptive Name"="Search FlexRay Cycle Count Min", "Data Type"=0, "Command"="SEAR:TRIG:FLXR:CMIN", "Access"=2, "Range Table"="rsscope_rngFlexRayCycleMinMax", "Read Callback"="rsscope_FormatSearchNameInt32_ReadCallback.vi", "Write Callback"="rsscope_FormatSearchNameInt32_WriteCallback.vi", "Supported Models"="", "Instrument Options"="", "Flags"=0, "Help"="Specifies a cycle count - the number of the current FlexRay cycle - or sets the start value of an cycle count range.\n\nAvailable Repeated Capabilities:\nNone\n\nRemote-control command(s):\nSEARch:TRIGger:FLXRay:CMIN"}, {"Level"=4, "Class Only"=FALSE, "Identifier"="RSSCOPE_ATTR_SEARCH_FLEXRAY_CYCLE_COUNT_MAX", "Descriptive Name"="Search FlexRay Cycle Count Max", "Data Type"=0, "Command"="SEAR:TRIG:FLXR:CMAX", "Access"=2, "Range Table"="rsscope_rngFlexRayCycleMinMax", "Read Callback"="rsscope_FormatSearchNameInt32_ReadCallback.vi", "Write Callback"="rsscope_FormatSearchNameInt32_WriteCallback.vi", "Supported Models"="", "Instrument Options"="", "Flags"=0, "Help"="Sets the end value of a cycle count range if the condition RSSCOPE_ATTR_SEARCH_FLEXRAY_CYCLE_COUNT_CONDITION is set to In range or Out of range.\n\nAvailable Repeated Capabilities:\nNone\n\nRemote-control command(s):\nSEARch:TRIGger:FLXRay:CMAX"}, {"Level"=4, "Class Only"=FALSE, "Identifier"="RSSCOPE_ATTR_SEARCH_FLEXRAY_CYCLE_COUNT_STEP", "Descriptive Name"="Search FlexRay Cycle Count Step", "Data Type"=0, "Command"="SEAR:TRIG:FLXR:CST", "Access"=2, "Range Table"="rsscope_rngFlexRayCycleStep", "Read Callback"="rsscope_FormatSearchNameInt32_ReadCallback.vi", "Write Callback"="rsscope_FormatSearchNameInt32_WriteCallback.vi", "Supported Models"="", "Instrument Options"="", "Flags"=0, "Help"="Specifies a step to search for each n-th cycle inside the given range. This allows for a specific search if slot multiplexing is used. The condition RSSCOPE_ATTR_SEARCH_FLEXRAY_CYCLE_COUNT_CONDITION must be set to In range or Out of range\n\nAvailable Repeated Capabilities:\nNone\n\nRemote-control command(s):\nSEARch:TRIGger:FLXRay:CSTep"}, {"Level"=4, "Class Only"=FALSE, "Identifier"="RSSCOPE_ATTR_SEARCH_FLEXRAY_DATA_POSITION_CONDITION", "Descriptive Name"="Search FlexRay Data Position Condition", "Data Type"=0, "Command"="SEAR:TRIG:FLXR:DPOP", "Access"=2, "Range Table"="RsScope_rngSearchFlexRayDataPositionCondition", "Read Callback"="rsscope_FormatSearchNameInt32_ReadCallback.vi", "Write Callback"="rsscope_FormatSearchNameInt32_WriteCallback.vi", "Supported Models"="", "Instrument Options"="", "Flags"=0, "Help"="Sets the operator for the data position. You can defined an exact position, or a position range.\n\nAvailable Repeated Capabilities:\nNone\n\nRemote-control command(s):\nSEARch:TRIGger:FLXRay:DPOPerator"}, {"Level"=4, "Class Only"=FALSE, "Identifier"="RSSCOPE_ATTR_SEARCH_FLEXRAY_DATA_POSITION_MIN", "Descriptive Name"="Search FlexRay Data Position Min", "Data Type"=0, "Command"="SEAR:TRIG:FLXR:DPOS", "Access"=2, "Range Table"="RsScope_rngSearchFlexRayDataPositionMinMax", "Read Callback"="rsscope_FormatSearchNameInt32_ReadCallback.vi", "Write Callback"="rsscope_FormatSearchNameInt32_WriteCallback.vi", "Supported Models"="", "Instrument Options"="", "Flags"=0, "Help"="Sets the number of data bytes to be skipped after start of the payload segment.\n\nAvailable 
